vi "Configure PKCE.vi"(7 "Use PKCE? (T)":bool=TRUE, 8 "error in":errorcluster, 11 "Oauth2 in":refnum<class "Oauth2.lvclass">) -> (0 "error out":errorcluster, 3 "Oauth2":refnum<class "Oauth2.lvclass">)   [LabVIEW 2013, in "Oauth2.lvclass"]
uses:
  Oauth2.lvclass
  OAuthToken/OAuth2 Token Element -- enum.ctl
  Oauth2.lvclass/Oauth2.ctl
  <vilib>/LabVIEW Open Source Project/OpenSerializer.Base64/Base64_CharSet.vi
  OAuthToken/OAuthAccessToken.lvclass
  <vilib>/LabVIEW Open Source Project/Unicity/RandomStringGenerator/RandomStringGenerator.lvclass
  <vilib>/LabVIEW Open Source Project/OpenSerializer.Base64/Serializer.Base64.lvclass
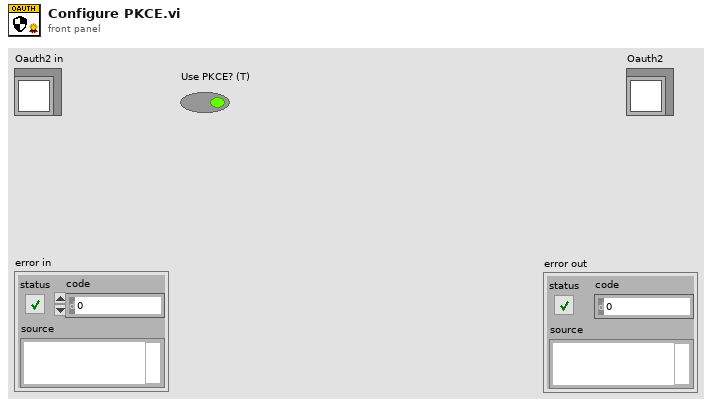
[diagram p1: front panel]
types:
  T1 = typedef "OAuthAccessToken.lvclass/OAuth2 Token Element -- enum.ctl" = enum16{"client_id", "client_secret", "response_type", "scope", "redirect_uri", "error", "error_description", "error_uri", "grant_type", "code", "access_token", "token_type", "expires_in", "username", "password", "refresh_token", "code_challenge", "code_challenge_method", "endpoint element"}
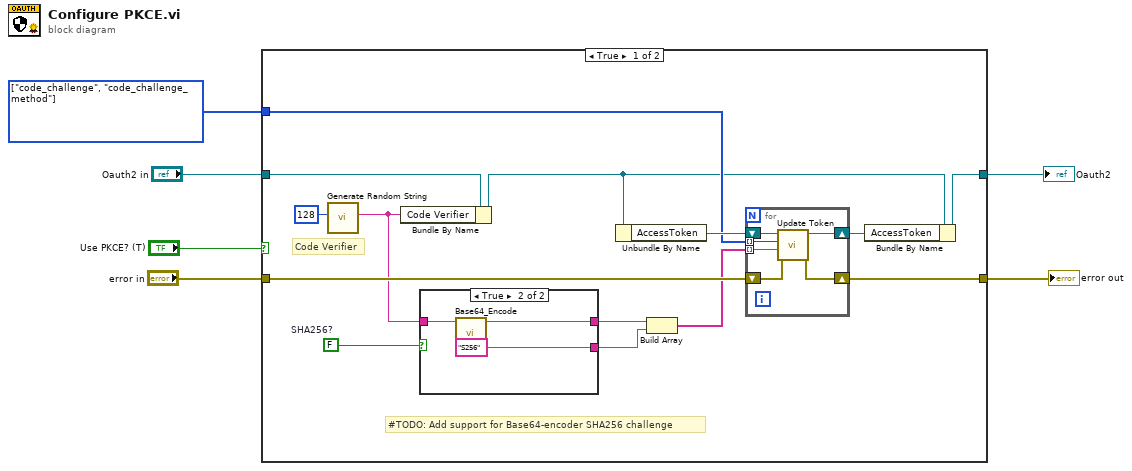
[diagram p0: block diagram]
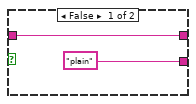
[diagram p2: hidden frame]
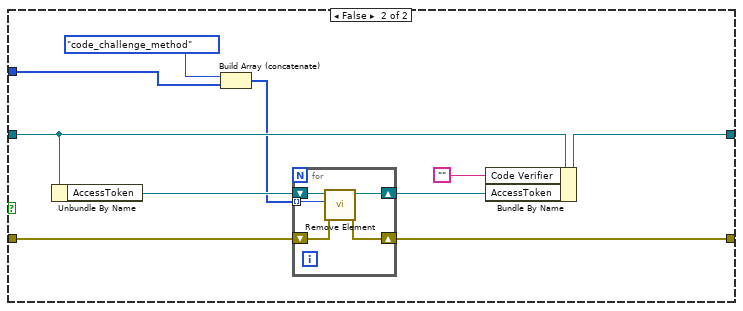
[diagram p3: hidden frame]
diagram:
  w5 = T1[] [enum."code_challenge", enum."code_challenge_method"] items=["client_id", "client_secret", "response_type", "scope", "redirect_uri", "error", "error_description", "error_uri", "grant_type", "code", "access_token", "token_type", "expires_in", "username", "password", "refresh_token", "code_challenge", "code_challenge_method", "endpoint element"]
  n1 = case shown="True" "Use PKCE? (T)" {
    tunnel: [w19 w40] -> w6
    tunnel: w5 -> [w17 w33]
    tunnel: [w16 w38] -> w4
    tunnel: "Oauth2 in" -> [w12 w37]
    tunnel: "error in" -> [w15 w36]
    frame True {
      w9 = FALSE  # SHA256?
      # "#TODO: Add support for Base64-encoder SHA256 challenge"
      # "Code Verifier"
      n2 = call <vilib>:"Generate Random String.vi"("String Length (32)"=u32 128) -> ("Random String"=w10:string)  [unwired: 10 in]
      n3 = Bundle By Name(cluster=w12, "Code Verifier"=w10) -> (w11:refnum<class "Oauth2.lvclass">)
      n4 = case shown="True" w9 {
        tunnel: [w22 w25] -> w7
        tunnel: w10 -> [w22 w24]
        tunnel: ["plain" ("argument") "S256" ("argument")] -> w8
        frame False {
        }
        frame True {
          n5 = call <vilib>:"Base64_Encode.vi"("String"=w24) -> ("Encoded String"=w25:string)  [unwired: 9 in, 1 out]
        }
      }
      n6 = Unbundle By Name(w11) -> ("AccessToken"=w20:refnum<class "OAuthAccessToken.lvclass">)
      n7 = Build Array(w7, w8) -> (w13:string[])
      n8 = for {
        tunnel: w13 -> [w30] mode=indexing
        shift-right: [w29] -> w18
        shift-left: w20 -> [w31]
        tunnel: w17 -> [w28] mode=indexing
        shift-right: [w26] -> w16
        shift-left: w15 -> [w27]
        n9 = call "Update Token.vi"("error in (no error)"=w27, "Value"=w30, "Token element"=w28, "OAuthAccessToken in"=w31) -> ("error out"=w26:errorcluster, "OAuthAccessToken out"=w29:refnum<class "OAuthAccessToken.lvclass">)  [unwired: 6 in]
      }
      n10 = Bundle By Name(cluster=w11, "AccessToken"=w18) -> (w19:refnum<class "Oauth2.lvclass">)
    }
    frame False {
      n11 = Unbundle By Name(w37) -> ("AccessToken"=w41:refnum<class "OAuthAccessToken.lvclass">)
      n12 = Build Array (concatenate)(OAuth2_Token_Element_--_enum."code_challenge_method" ("Token element"), w33) -> (w32:T1[])
      n13 = for {
        shift-right: [w45] -> w39
        shift-left: w41 -> [w46]
        tunnel: w32 -> [w42] mode=indexing
        shift-right: [w44] -> w38
        shift-left: w36 -> [w43]
        n14 = call "Remove Element.vi"("error in (no error)"=w43, "Token element"=w42, "OAuthAccessToken in"=w46) -> ("error out"=w44:errorcluster, "OAuthAccessToken out"=w45:refnum<class "OAuthAccessToken.lvclass">)  [unwired: 6 in, 1 out]
      }
      n15 = Bundle By Name(cluster=w37, "Code Verifier"="", "AccessToken"=w39) -> (w40:refnum<class "Oauth2.lvclass">)
    }
  }
  "Oauth2" <- w6
  "error out" <- w4
